vi "KH TURCK ETHERNETIP IOL Status.vi"(8 "Data_IO":T2, 11 "DataItem.Data":u8[](array[numeric])) -> (3 "Status":T1)   [LabVIEW 2021]
uses:
  KH TURCK ETHERNETIP TDef Enum IOL Data.ctl
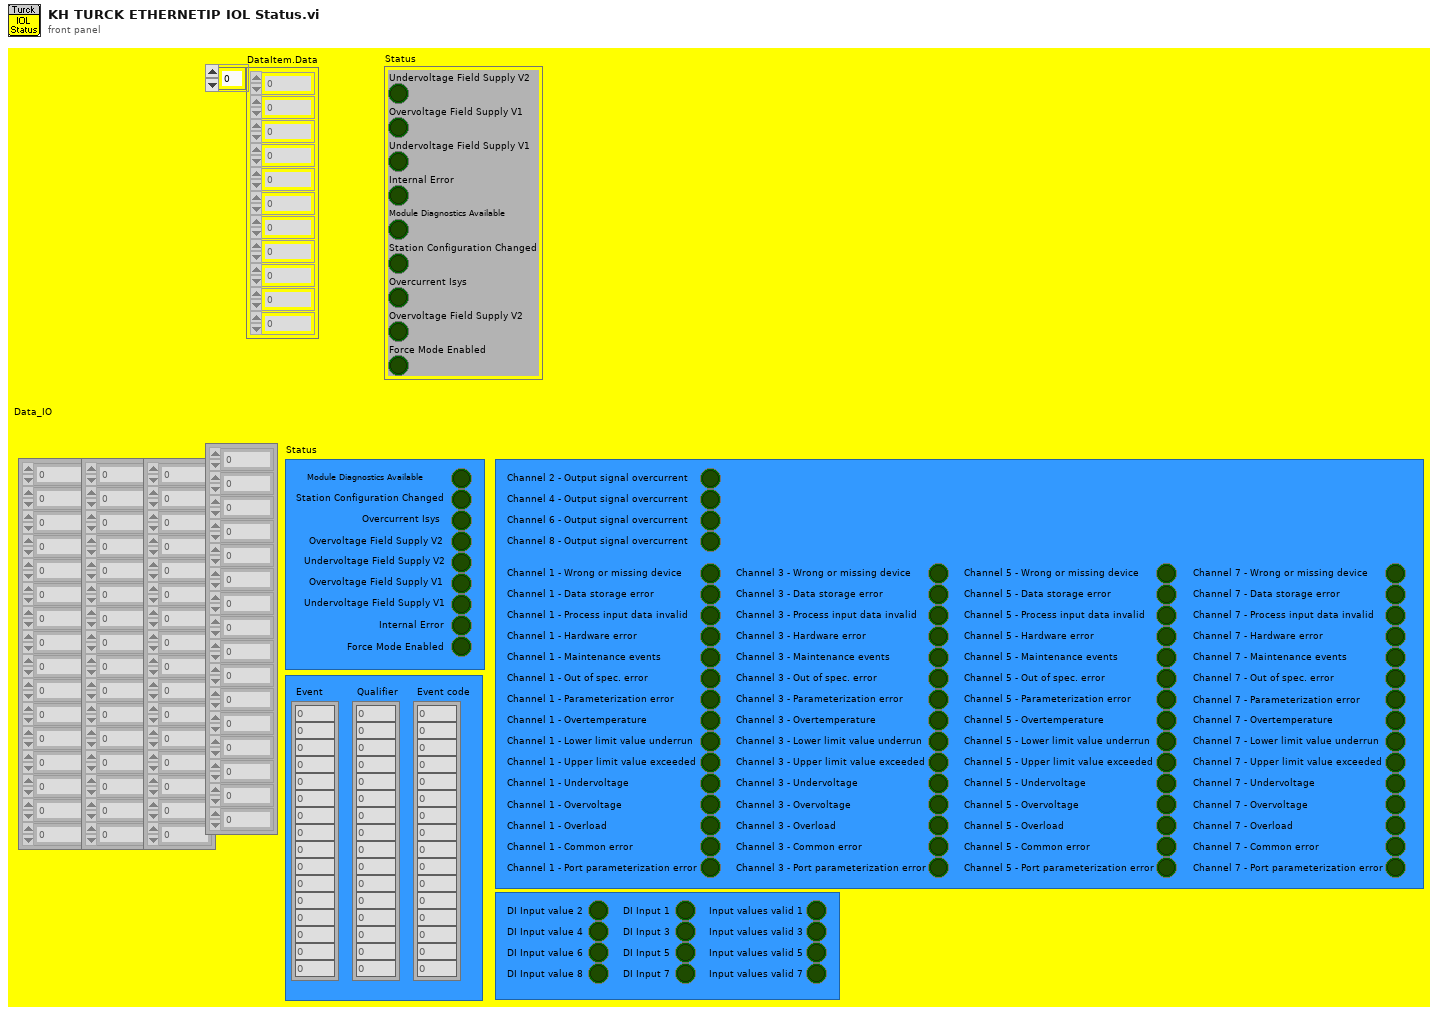
[diagram p1: front panel]
types:
  T1 = cluster{"Undervoltage Field Supply V2":bool, "Overvoltage Field Supply V1":bool, "Undervoltage Field Supply V1":bool, "Internal Error":bool, "Module Diagnostics Available":bool, "Station Configuration Changed":bool, "Overcurrent Isys":bool, "Overvoltage Field Supply V2":bool, "Force Mode Enabled":bool}
  T2 = typedef "KH TURCK ETHERNETIP TDef Enum IOL Data.ctl" = cluster{"Data_Port1":u16[], "Data_Port3":u16[], "Data_Port5":u16[], "Data_Port7":u16[], "Status":cluster{"Undervoltage Field Supply V2":bool, "Overvoltage Field Supply V1":bool, "Undervoltage Field Supply V1":bool, "Internal Error":bool, "Module Diagnostics Available":bool, "Station Configuration Changed":bool, "Overcurrent Isys":bool, "Overvoltage Field Supply V2":bool, "Force Mode Enabled":bool}, "Diagnostics":cluster{"Channel 2 - Output signal overcurrent":bool, "Channel 4 - Output signal overcurrent":bool, "Channel 6 - Output signal overcurrent":bool, "Channel 8 - Output signal overcurrent":bool, "Channel 1 - Wrong or missing device":bool, "Channel 3 - Wrong or missing device":bool, "Channel 5 - Wrong or missing device":bool, "Channel 7 - Wrong or missing device":bool, "Channel 1 - Data storage error":bool, "Channel 3 - Data storage error":bool, "Channel 5 - Data storage error":bool, "Channel 7 - Data storage error":bool, "Channel 1 - Process input data invalid":bool, "Channel 3 - Process input data invalid":bool, "Channel 5 - Process input data invalid":bool, "Channel 7 - Process input data invalid":bool, "Channel 1 - Hardware error":bool, "Channel 3 - Hardware error":bool, "Channel 5 - Hardware error":bool, "Channel 7 - Hardware error":bool, "Channel 1 - Maintenance events":bool, "Channel 3 - Maintenance events":bool, "Channel 5 - Maintenance events":bool, "Channel 7 - Maintenance events":bool, "Channel 1 - Out of spec. error":bool, "Channel 3 - Out of spec. error":bool, "Channel 5 - Out of spec. error":bool, "Channel 7 - Out of spec. error":bool, "Channel 1 - Parameterization error":bool, "Channel 3 - Parameterization error":bool, "Channel 5 - Parameterization error":bool, "Channel 1 - Overtemperature":bool, "Channel 3 - Overtemperature":bool, "Channel 5 - Overtemperature":bool, "Channel 7 - Overtemperature":bool, "Channel 1 - Lower limit value underrun":bool, "Channel 3 - Lower limit value underrun":bool, "Channel 5 - Lower limit value underrun":bool, "Channel 7 - Lower limit value underrun":bool, "Channel 1 - Upper limit value exceeded":bool, "Channel 3 - Upper limit value exceeded":bool, "Channel 5 - Upper limit value exceeded":bool, "Channel 7 - Upper limit value exceeded":bool, "Channel 1 - Undervoltage":bool, "Channel 3 - Undervoltage":bool, "Channel 5 - Undervoltage":bool, "Channel 7 - Undervoltage":bool, "Channel 1 - Overvoltage":bool, "Channel 3 - Overvoltage":bool, "Channel 5 - Overvoltage":bool, "Channel 7 - Overvoltage":bool, "Channel 1 - Overload":bool, "Channel 3 - Overload":bool, "Channel 5 - Overload":bool, "Channel 7 - Overload":bool, "Channel 1 - Common error":bool, "Channel 3 - Common error":bool, "Channel 5 - Common error":bool, "Channel 7 - Common error":bool, "Channel 1 - Port parameterization error":bool, "Channel 3 - Port parameterization error":bool, "Channel 5 - Port parameterization error":bool, "Channel 7 - Parameterization error":bool, "Channel 7 - Port parameterization error":bool}, "Events":cluster{"Event":u8[], "Qualifier":u8[], " Event code":u16[]}, "DXP":cluster{"DI Input value 2":bool, "DI Input value 4":bool, "DI Input value 6":bool, "DI Input value 8":bool, "DI Input 1":bool, "DI Input 3":bool, "DI Input 5":bool, "DI Input 7":bool, "Input values valid 1":bool, "Input values valid 3":bool, "Input values valid 5":bool, "Input values valid 7":bool}}
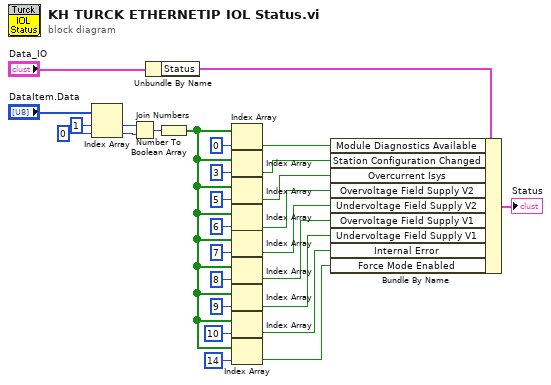
[diagram p0: block diagram]
diagram:
  n1 = Index Array(array="DataItem.Data", index #1=1 ("index"), index #2=0 ("index")) -> (element #1=w27:u8, element #2=w1:u8)
  n2 = Join Numbers(hi=w27, lo=w1) -> ((hi.lo)=w26:u16)
  n3 = Unbundle By Name("Data_IO") -> ("Status"=w25:T1)
  n4 = Number To Boolean Array(number=w26) -> (Boolean array=w12:bool[])
  n5 = Index Array(array=w12, index=0) -> (element=w20:bool)
  n6 = Index Array(array=w12, index=3) -> (element=w11:bool)
  n7 = Index Array(array=w12, index=5) -> (element=w10:bool)
  n8 = Index Array(array=w12, index=6) -> (element=w9:bool)
  n9 = Index Array(array=w12, index=7) -> (element=w8:bool)
  n10 = Index Array(array=w12, index=8) -> (element=w7:bool)
  n11 = Index Array(array=w12, index=9) -> (element=w6:bool)
  n12 = Index Array(array=w12, index=10) -> (element=w5:bool)
  n13 = Index Array(array=w12, index=14) -> (element=w4:bool)
  n14 = Bundle By Name(cluster=w25, "Module Diagnostics Available"=w20, "Station Configuration Changed"=w11, "Overcurrent Isys"=w10, "Overvoltage Field Supply V2"=w9, "Undervoltage Field Supply V2"=w8, "Overvoltage Field Supply V1"=w7, "Undervoltage Field Supply V1"=w6, "Internal Error"=w5, "Force Mode Enabled"=w4) -> (→"Status":T1)
